vi "DXFGraghicDisplay.vi"(9 "Index":i32, 10 "CADIn":T1, 11 "empty picture":picture) -> (3 "new picture":picture)   [LabVIEW 2014]
uses:
  Button_ctl/TeachDataHandle.ctl
  Button_ctl/TeachDataDispose.ctl
  <vilib>/Utility/miscctls.llb/LVPointTypeDef.ctl
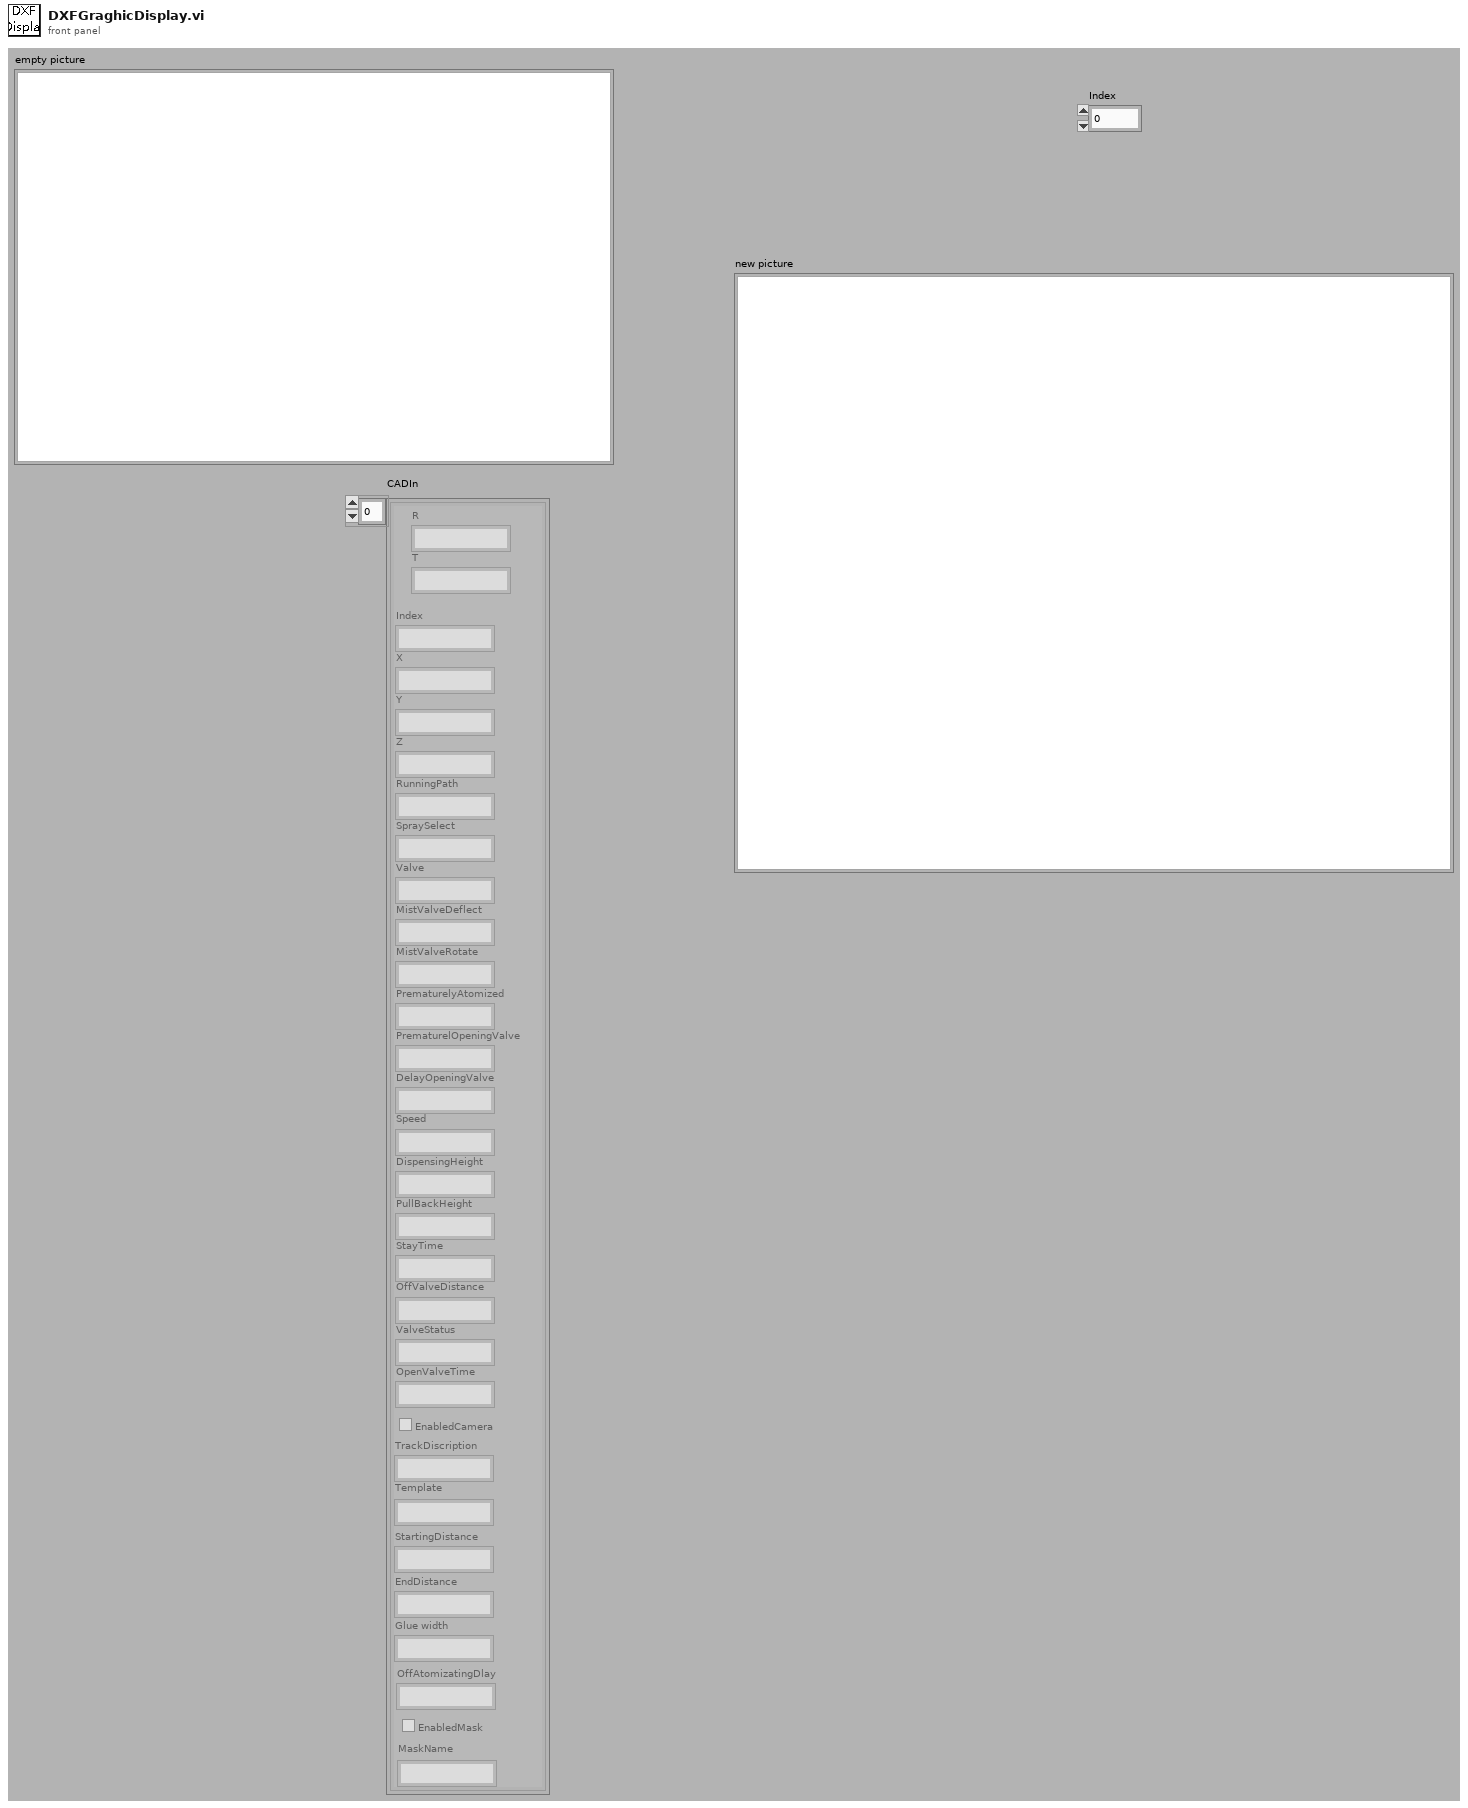
[diagram p1: front panel]
types:
  T1 = typedef "TeachDataHandle.ctl" = T2[]
  T2 = typedef "TeachDataDispose.ctl" = cluster{"Index":string, "X":string, "Y":string, "Z":string, "RunningPath":string, "SpraySelect":string, "Valve":string, "MistValveDeflect":string, "MistValveRotate":string, "PrematurelyAtomized":string, "PrematurelOpeningValve":string, "DelayOpeningValve":string, "Speed":string, "DispensingHeight":string, "PullBackHeight":string, "StayTime":string, "OffValveDistance":string, "ValveStatus":string, "OpenValveTime":string, "CameraOperating":bool, "TrackDiscription":string, "Template":string, "StartingDistance":string, "EndDistance":string, "Glue width":string, "OffAtomizatingDlay":string, "EnabledMask":bool, "MaskName":string, "T":string, "R":string}
  T3 = typedef "LVPointTypeDef.ctl" = cluster{"Horizontal":i16, "Vertical":i16}
  T4 = cluster{"Width":u16, "Style":enum32{"Solid", "Dash", "Dot", "DashDot", "DashDotDot"}}
  T5 = cluster{"Width":i32, "Style":enum32{"Solid", "Dash", "Dot", "DashDot", "DashDotDot"}}
  T6 = typedef "LVBoundsTypeDef.ctl" = cluster{"Width":u32, "Height":u32}
  T7 = cluster{"X":dbl, dbl, "X":dbl, "Y":dbl, "X":dbl, dbl}
  T8 = cluster{"Xc":dbl, "Yc":dbl, "R1":dbl, "StA":dbl, "EnA":dbl, "TravelAngle":dbl}
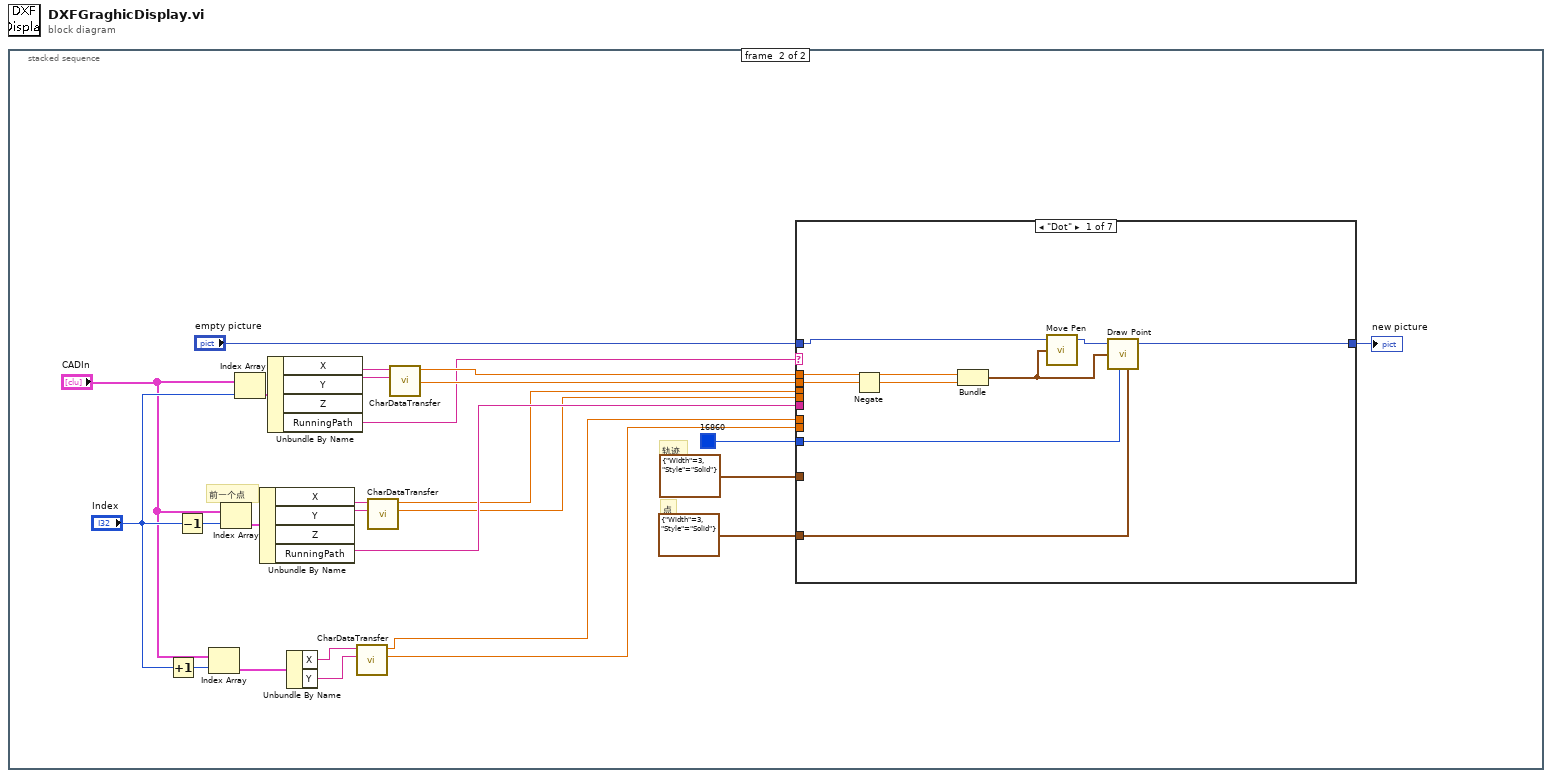
[diagram p0: block diagram]
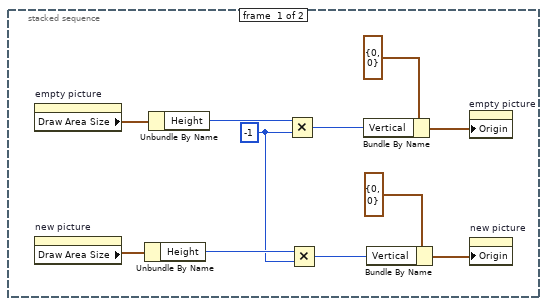
[diagram p2: hidden frame]
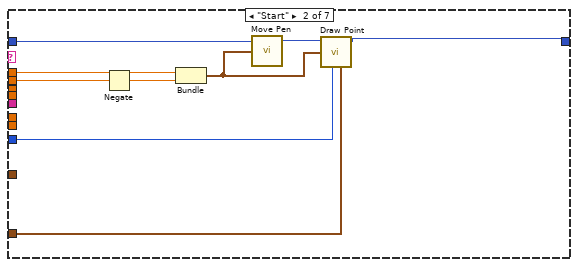
[diagram p3: hidden frame]
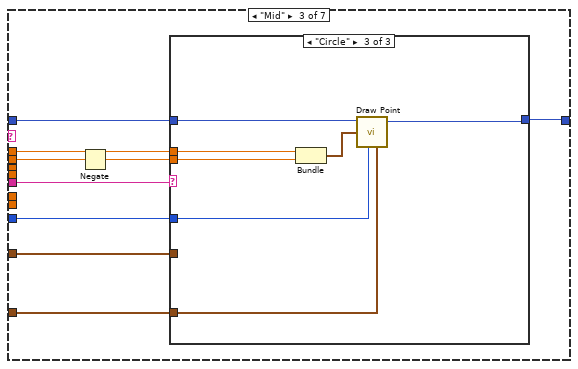
[diagram p4: hidden frame]
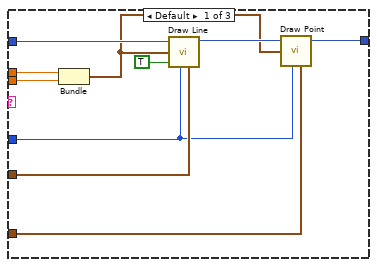
[diagram p5: hidden frame]
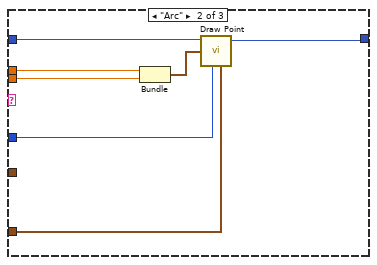
[diagram p6: hidden frame]
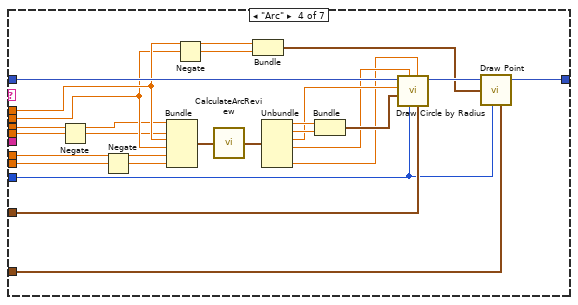
[diagram p7: hidden frame]
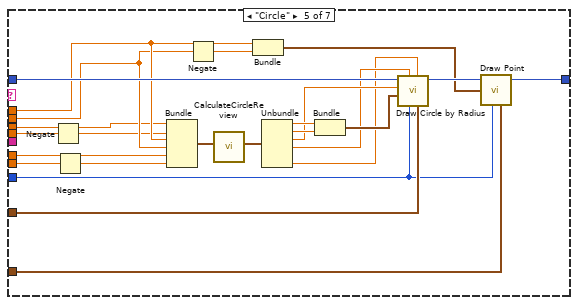
[diagram p8: hidden frame]
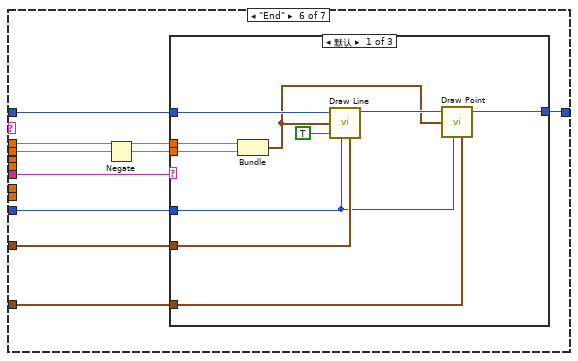
[diagram p9: hidden frame]
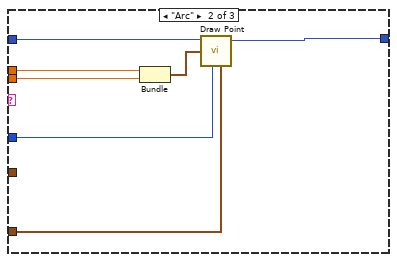
[diagram p10: hidden frame]
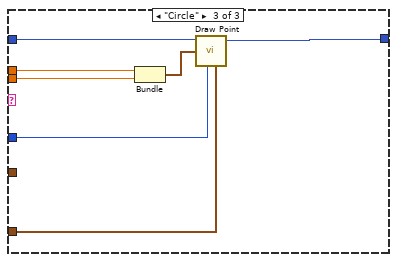
[diagram p11: hidden frame]
diagram:
  n1 = stacked-sequence {
    frame #0 {
      w4 = -1 ("y")
      n2 = property on="empty picture" class="Pict"() -> ("Draw Area Size"=w11:T6)  [unwired: 2 in, 2 out]
      n3 = property on="new picture" class="Pict"() -> ("Draw Area Size"=w6:T6)  [unwired: 2 in, 2 out]
      n4 = Unbundle By Name(w6) -> ("Height"=w5:u32)
      n5 = Unbundle By Name(w11) -> ("Height"=w10:u32)
      n6 = Multiply(x=w10, y=w4) -> (x*y=w8:u32)
      n7 = Multiply(x=w5, y=w4) -> (x*y=w3:u32)
      n8 = Bundle By Name(cluster=T3 {"Horizontal"=0, "Vertical"=0} ("原点"), "Vertical"=w8) -> (w7:T3)
      n9 = Bundle By Name(cluster=T3 {"Horizontal"=0, "Vertical"=0} ("原点"), "Vertical"=w3) -> (w1:T3)
      n10 = property on="empty picture" class="Pict"("Origin"=w7) -> ()  [unwired: 2 in, 2 out]
      n11 = property on="new picture" class="Pict"("Origin"=w1) -> ()  [unwired: 2 in, 2 out]
    }
    frame #1 {
      # "前一个点"
      # "点"
      # "轨迹"
      n12 = Increment(x="Index") -> (x+1=w33:i32)
      n13 = Decrement(x="Index") -> (x-1=w34:i32)
      n14 = Index Array(array="CADIn", index=w33) -> (element=w16:T2)
      n15 = Index Array(array="CADIn", index=w34) -> (element=w22:T2)
      n16 = Index Array(array="CADIn", index="Index") -> (element=w28:T2)
      n17 = Unbundle By Name(w22) -> ("X"=w20:string, "Y"=w19:string, "RunningPath"=w21:string)  [unwired: 1 out]
      n18 = Unbundle By Name(w28) -> ("X"=w27:string, "Y"=w26:string, "RunningPath"=w23:string)  [unwired: 1 out]
      n19 = Unbundle By Name(w16) -> ("X"=w15:string, "Y"=w14:string)
      n20 = call "CharDataTransfer.vi"("Y"=w14, "X"=w15) -> ("Y"=w12:dbl, "X"=w13:dbl)  [unwired: 3 in, 1 out]
      n21 = call "CharDataTransfer.vi"("Y"=w19, "X"=w20) -> ("Y"=w17:dbl, "X"=w18:dbl)  [unwired: 3 in, 1 out]
      n22 = call "CharDataTransfer.vi"("Y"=w26, "X"=w27) -> ("Y"=w24:dbl, "X"=w25:dbl)  [unwired: 3 in, 1 out]
      n23 = case shown="\"Dot\"" w23 {
        tunnel: "empty picture" -> [w41 w49 w64 w110 w134 w145 w170]
        tunnel: [w46 w51 w61 w101 w125 w142 w170] -> w30
        tunnel: u32 16860 ("color(black)") -> [w44 w55 w63 w99 w123 w144 _]
        tunnel: T5 {"Width"=3, "Style"=enum."Solid"} ("pen") -> [_ _ w62 w109 w133 w143 _]
        tunnel: T4 {"Width"=3, "Style"=enum."Solid"} ("pen") -> [w45 w54 w60 w98 w122 w141 _]
        tunnel: w25 -> [w43 w53 w59 w97 w121 w140 _]
        tunnel: w24 -> [w42 w52 w58 w96 w120 w139 _]
        tunnel: w21 -> [_ _ w57 _ _ w138 _]
        tunnel: w18 -> [_ _ _ w95 w119 _ _]
        tunnel: w17 -> [_ _ _ w94 w118 _ _]
        tunnel: w13 -> [_ _ _ w93 w117 _ _]
        tunnel: w12 -> [_ _ _ w92 w116 _ _]
        frame "Dot" {
          n24 = Negate(x=w42) -> (-x=w38:dbl)
          n25 = Bundle("X"=w43, w38) -> (w39:cluster{"X":dbl, dbl})  [unwired: 1 in]
          n26 = call <vilib>:"Move Pen.vi"("new position"=w39, "picture"=w41) -> ("new picture"=w40:picture)  [unwired: 3 in]
          n27 = call <vilib>:"Draw Point.vi"("picture"=w40, "point(x,y)"=w39, "color(black)"=w44, "pen"=w45) -> ("new picture"=w46:picture)  [unwired: 5 in]
        }
        frame "Start" {
          n28 = Negate(x=w52) -> (-x=w47:dbl)
          n29 = Bundle("X"=w53, w47) -> (w48:cluster{"X":dbl, dbl})  [unwired: 1 in]
          n30 = call <vilib>:"Move Pen.vi"("new position"=w48, "picture"=w49) -> ("new picture"=w50:picture)  [unwired: 3 in]
          n31 = call <vilib>:"Draw Point.vi"("picture"=w50, "point(x,y)"=w48, "color(black)"=w55, "pen"=w54) -> ("new picture"=w51:picture)  [unwired: 5 in]
        }
        frame "Mid" {
          n32 = Negate(x=w58) -> (-x=w56:dbl)
          n33 = case shown="\"Circle\"" w57 {
            tunnel: w64 -> [w74 w78 w85]
            tunnel: w59 -> [w73 w80 w87]
            tunnel: w56 -> [w72 w79 w86]
            tunnel: w63 -> [w66 w76 w83]
            tunnel: w62 -> [w70 _ _]
            tunnel: [w67 w77 w84] -> w61
            tunnel: w60 -> [w65 w75 w82]
            frame Default {
              n34 = Bundle("X"=w73, w72) -> (w68:cluster{"X":dbl, dbl})  [unwired: 1 in]
              n35 = call <vilib>:"Draw Line.vi"("picture"=w74, "end point"=w68, "absolute coordinates?(T)"=TRUE, "color(black)"=w66, "pen"=w70) -> ("new picture"=w69:picture)  [unwired: 4 in]
              n36 = call <vilib>:"Draw Point.vi"("picture"=w69, "point(x,y)"=w68, "color(black)"=w66, "pen"=w65) -> ("new picture"=w67:picture)  [unwired: 5 in]
            }
            frame "Arc" {
              n37 = Bundle("X"=w80, w79) -> (w81:cluster{"X":dbl, dbl})  [unwired: 1 in]
              n38 = call <vilib>:"Draw Point.vi"("picture"=w78, "point(x,y)"=w81, "color(black)"=w76, "pen"=w75) -> ("new picture"=w77:picture)  [unwired: 5 in]
            }
            frame "Circle" {
              n39 = Bundle("X"=w87, w86) -> (w88:cluster{"X":dbl, dbl})  [unwired: 1 in]
              n40 = call <vilib>:"Draw Point.vi"("picture"=w85, "point(x,y)"=w88, "color(black)"=w83, "pen"=w82) -> ("new picture"=w84:picture)  [unwired: 5 in]
            }
          }
        }
        frame "Arc" {
          n41 = Negate(x=w94) -> (-x=w89:dbl)
          n42 = Negate(x=w92) -> (-x=w90:dbl)
          n43 = Bundle("X"=w95, w89, "X"=w97, "Y"=w96, "X"=w93, w90) -> (w112:T7)  [unwired: 1 in]
          n44 = Negate(x=w96) -> (-x=w91:dbl)
          n45 = call "CalculateArcReview.vi"("Input"=w112) -> ("Output"=w111:T8)  [unwired: 4 in]
          n46 = Bundle("X"=w97, w91) -> (w100:cluster{"X":dbl, dbl})  [unwired: 1 in]
          n47 = Unbundle(w111) -> ("Xc"=w108:dbl, "Yc"=w107:dbl, "R1"=w105:dbl, "StA"=w104:dbl, "TravelAngle"=w103:dbl)  [unwired: 1 out]
          n48 = Bundle("Xc"=w108, "Yc"=w107) -> (w106:cluster{"Xc":dbl, "Yc":dbl})  [unwired: 1 in]
          n49 = call <vilib>:"Draw Circle by Radius.vi"("pen"=w109, "arc size(360)"=w103, "color(black)"=w99, "start angle(0)"=w104, "pixel center"=w106, "radius"=w105, "picture"=w110) -> ("new picture"=w102:picture)  [unwired: 4 in]
          n50 = call <vilib>:"Draw Point.vi"("picture"=w102, "point(x,y)"=w100, "color(black)"=w99, "pen"=w98) -> ("new picture"=w101:picture)  [unwired: 5 in]
        }
        frame "Circle" {
          n51 = Negate(x=w118) -> (-x=w114:dbl)
          n52 = Negate(x=w116) -> (-x=w113:dbl)
          n53 = Bundle("X"=w119, w114, "X"=w121, "Y"=w120, "X"=w117, w113) -> (w136:T7)  [unwired: 1 in]
          n54 = Negate(x=w120) -> (-x=w115:dbl)
          n55 = call "CalculateCircleReview.vi"("Input"=w136) -> ("Output"=w135:T8)  [unwired: 6 in]
          n56 = Bundle("X"=w121, w115) -> (w124:cluster{"X":dbl, dbl})  [unwired: 1 in]
          n57 = Unbundle(w135) -> ("Xc"=w132:dbl, "Yc"=w131:dbl, "R1"=w129:dbl, "StA"=w128:dbl, "TravelAngle"=w127:dbl)  [unwired: 1 out]
          n58 = Bundle("Xc"=w132, "Yc"=w131) -> (w130:cluster{"Xc":dbl, "Yc":dbl})  [unwired: 1 in]
          n59 = call <vilib>:"Draw Circle by Radius.vi"("pen"=w133, "arc size(360)"=w127, "color(black)"=w123, "start angle(0)"=w128, "pixel center"=w130, "radius"=w129, "picture"=w134) -> ("new picture"=w126:picture)  [unwired: 4 in]
          n60 = call <vilib>:"Draw Point.vi"("picture"=w126, "point(x,y)"=w124, "color(black)"=w123, "pen"=w122) -> ("new picture"=w125:picture)  [unwired: 5 in]
        }
        frame "End" {
          n61 = Negate(x=w139) -> (-x=w137:dbl)
          n62 = case shown="默认" w138 {
            tunnel: w145 -> [w155 w162 w169]
            tunnel: w140 -> [w149 w159 w165]
            tunnel: w137 -> [w148 w158 w164]
            tunnel: w144 -> [w151 w161 w168]
            tunnel: w143 -> [w153 _ _]
            tunnel: [w146 w156 w163] -> w142
            tunnel: w141 -> [w150 w160 w167]
            frame Default {
              n63 = Bundle("X"=w149, w148) -> (w147:cluster{"X":dbl, dbl})  [unwired: 1 in]
              n64 = call <vilib>:"Draw Line.vi"("picture"=w155, "end point"=w147, "absolute coordinates?(T)"=TRUE, "color(black)"=w151, "pen"=w153) -> ("new picture"=w152:picture)  [unwired: 4 in]
              n65 = call <vilib>:"Draw Point.vi"("picture"=w152, "point(x,y)"=w147, "color(black)"=w151, "pen"=w150) -> ("new picture"=w146:picture)  [unwired: 5 in]
            }
            frame "Arc" {
              n66 = Bundle("X"=w159, w158) -> (w157:cluster{"X":dbl, dbl})  [unwired: 1 in]
              n67 = call <vilib>:"Draw Point.vi"("picture"=w162, "point(x,y)"=w157, "color(black)"=w161, "pen"=w160) -> ("new picture"=w156:picture)  [unwired: 5 in]
            }
            frame "Circle" {
              n68 = Bundle("X"=w165, w164) -> (w166:cluster{"X":dbl, dbl})  [unwired: 1 in]
              n69 = call <vilib>:"Draw Point.vi"("picture"=w169, "point(x,y)"=w166, "color(black)"=w168, "pen"=w167) -> ("new picture"=w163:picture)  [unwired: 5 in]
            }
          }
        }
        frame Default {
        }
      }
      "new picture" <- w30
    }
  }
